vi "Request.vi"(0 "Destination Address":u8 format="%.0x", 5 "Source Address":u8=27, 7 "PGN":u32 format="%.0x") -> (4 "Arb ID":u32 format="%.0x", 6 "Expected Return Arb ID":u32 format="%.0x", 8 "Data":u8[](array[numeric]) format="%.0x")   [LabVIEW 2019, in "J1939 Utilities.lvlib"]
uses:
  J1939 Utilities.lvlib
  Types/PGN Fields Cluster.ctl
  Convert J1939 ID to CAN Arb ID.vi
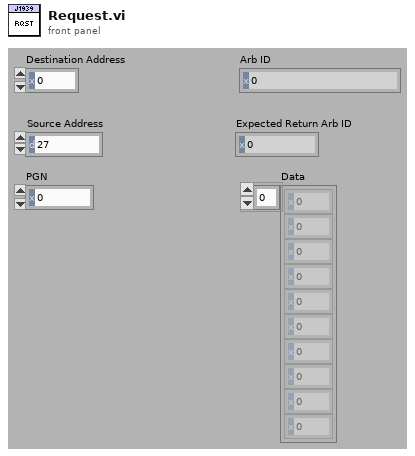
[diagram p1: front panel]
types:
  T1 = typedef "J1939 Utilities.lvlib/PGN Fields Cluster.ctl" = cluster{"Reserved Bit":u8, "Data page":u8, "PDU Format":u8, "PDU Specific":u8}
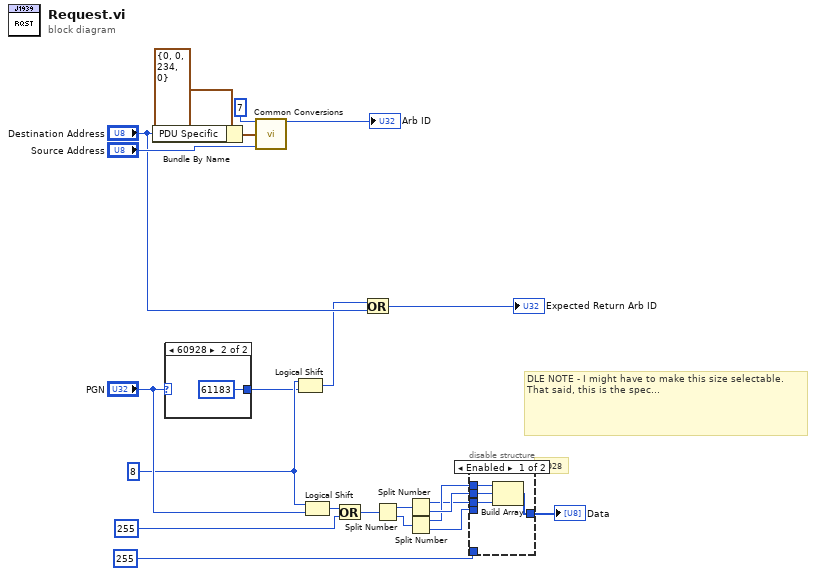
[diagram p0: block diagram]
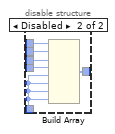
[diagram p3: hidden frame]
diagram:
  w5 = i8 8 ("y")
  # "DLE NOTE - I might have to make this size selectable.  That said, this is the spec..."
  # "60928"
  n1 = Bundle By Name(cluster=T1 {"Reserved Bit"=0, "Data page"=0, "PDU Format"=234, "PDU Specific"=0} ("PGN Fields"), "PDU Specific"="Destination Address") -> (w21:T1)
  n2 = case shown="60928" "PGN" {
    selector: "PGN" -> [w23 _]
    tunnel: [w23 u32 61183 ("PGN")] -> w4
    frame Default {
    }
    frame 60928 {
    }
  }
  n3 = call-poly "Common Conversions.vi"("Priority"=u8 7, "PGN Fields"=w21, "Source Address"="Source Address") -> ("ID"=→"Arb ID":u32)  [unwired: 2 in, 10 out]
  n4 = Logical Shift(y=w5, x=w4) -> (x << y=w3:u32)
  n5 = Logical Shift(y=w5, x="PGN") -> (x << y=w2:u32)
  n6 = Or(x=w2, y=u32 255 ("x")) -> (x .or. y?=w16:u32)
  n7 = Or(x=w3, y="Destination Address") -> (x .or. y?=→"Expected Return Arb ID":u32)
  n8 = Split Number(x=w16) -> (hi(x)=w15:u16, lo(x)=w14:u16)
  n9 = Split Number(x=w15) -> (hi(x)=w7:u8, lo(x)=w13:u8)
  n10 = Split Number(x=w14) -> (hi(x)=w8:u8, lo(x)=w12:u8)
  n11 = disable-structure shown="Enabled" {
    disable-tunnel: w13 -> [w28 w34]
    disable-tunnel: w12 -> [_ w33]
    disable-tunnel: u8 255 ("x") -> [_ w32]
    disable-tunnel: [w27 w31] -> w9
    disable-tunnel: w8 -> [w26 w30]
    disable-tunnel: w7 -> [w25 w29]
    frame Enabled {
      n12 = Build Array(w26, w28, w25) -> (w27:u8[])
    }
    frame Disabled {
      n13 = Build Array(w30, w34, w29, w33, w32, w32, w32, w32) -> (w31:u8[])
    }
  }
  "Data" <- w9
